vi "Change State.vi"(8 "error in (no error)":errorcluster, 10 "New State":T1=enum."Hover", 11 "Filled Text Fields Actor in":refnum<class "Filled Text Fields Actor.lvclass">) -> (0 "error out":errorcluster, 3 "Filled Text Fields Actor out":refnum<class "Filled Text Fields Actor.lvclass">)   [LabVIEW 2017, in "Filled Text Fields.lvlib" / "Filled Text Fields Actor.lvclass"]
uses:
  Filled Text Fields Actor.lvclass
  Filled Text Fields.States.ctl
  Filled Text Fields Actor.lvclass/Filled Text Fields Actor.ctl
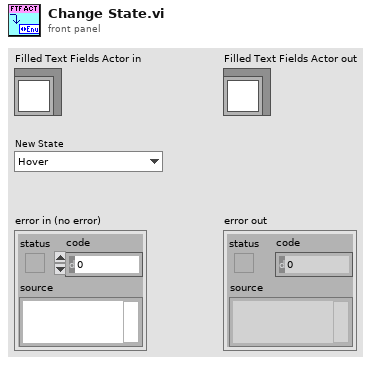
[diagram p1: front panel]
types:
  T1 = typedef "Filled Text Fields.lvlib/Filled Text Fields Actor.lvclass/Filled Text Fields.States.ctl" = enum16{"Inactive", "Activated", "Error", "Focused", "Hover", "Disabled", "Disabled and Grey out"}
  T2 = enum8{"Enabled", "Disabled", "Disabled and Grayed Out"}
  T3 = typedef "Theme.lvlib/Theme.Colors.lvclass/Colors.ctl" = cluster{"Main":cluster{"Primary":u32, "Primary Variant":u32, "Secondary":u32, "Secondary Varient":u32}, "Container":cluster{"BG":u32, "Hover":u32, "Focused":u32}, "Text":cluster{"Default":u32, "Error":u32}}
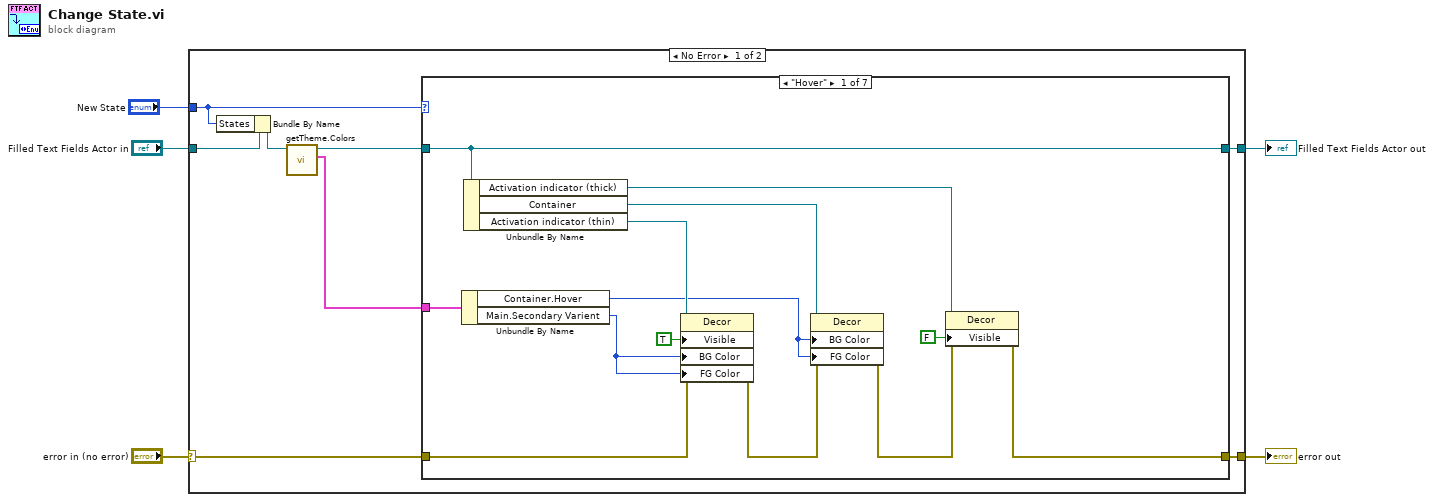
[diagram p0: block diagram]
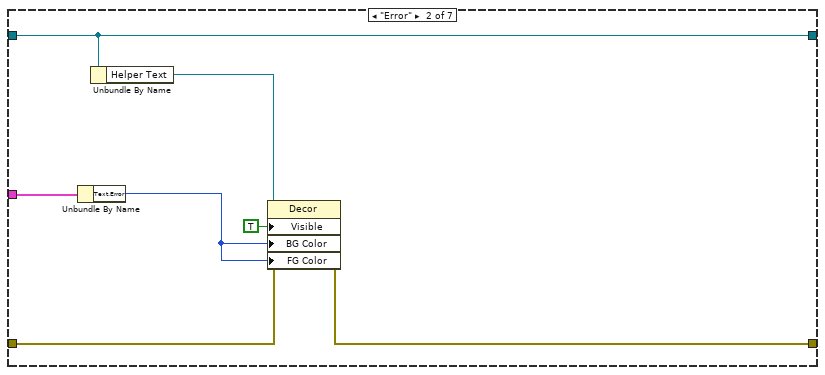
[diagram p2: hidden frame]
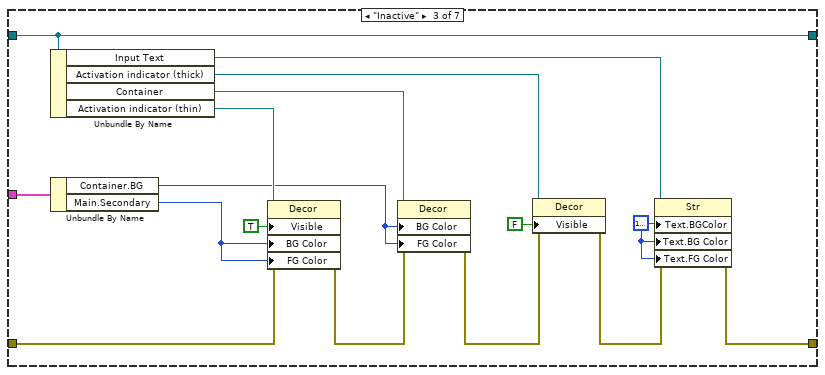
[diagram p3: hidden frame]
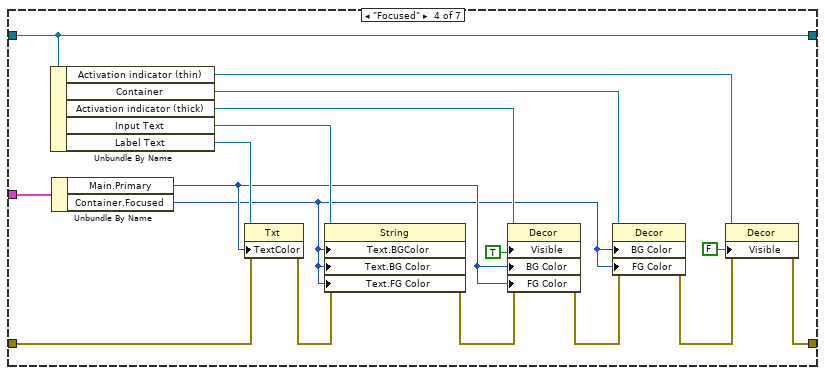
[diagram p4: hidden frame]
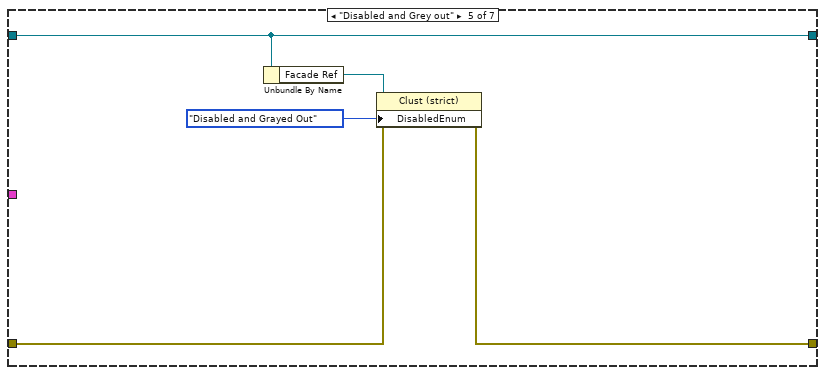
[diagram p5: hidden frame]
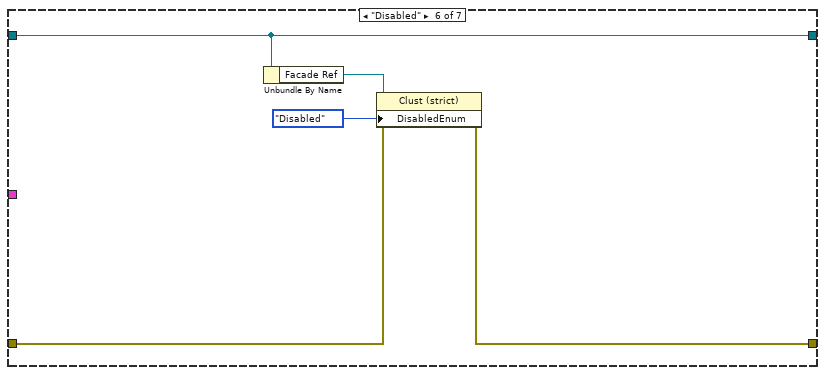
[diagram p6: hidden frame]
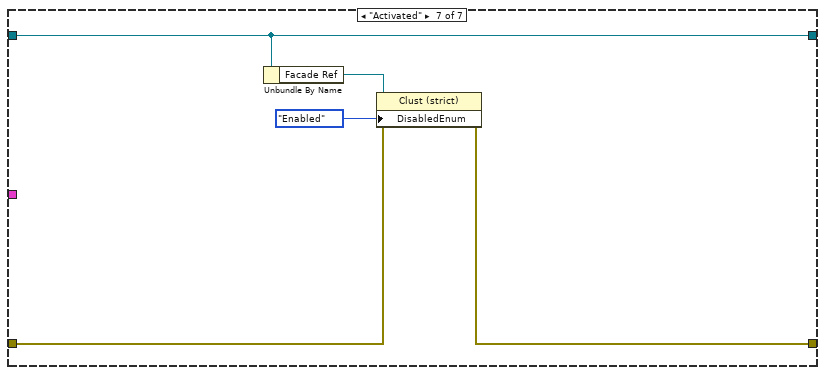
[diagram p7: hidden frame]
diagram:
  n1 = case shown="No Error" "error in (no error)" {
    selector: "error in (no error)" -> [w11 w83]
    tunnel: [w10 w83] -> w4
    tunnel: [w12 w82] -> w2
    tunnel: "Filled Text Fields Actor in" -> [w13 w82]
    tunnel: "New State" -> [w8 _]
    frame No Error {
      n2 = Bundle By Name(cluster=w13, "States"=w8) -> (w9:refnum<class "Filled Text Fields Actor.lvclass">)
      n3 = call "getTheme.Colors.vi"("Filled Text Fields Actor in"=w9) -> ("Colors"=w6:T3, "Filled Text Fields Actor out"=w7:refnum<class "Filled Text Fields Actor.lvclass">)  [unwired: 9 in]
      n4 = case shown="\"Hover\"" w8 {
        tunnel: w7 -> [w22 w32 w45 w62 w71 w76 w81]
        tunnel: [w22 w32 w45 w62 w71 w76 w81] -> w12
        tunnel: w11 -> [w21 w31 w44 w53 w68 w73 w78]
        tunnel: [w18 w29 w38 w59 w67 w72 w77] -> w10
        tunnel: w6 -> [w16 w28 w36 w52 _ _ _]
        frame "Hover" {
          n5 = Unbundle By Name(w16) -> ("Container.Hover"=w14:u32, "Main.Secondary Varient"=w15:u32)
          n6 = Unbundle By Name(w22) -> ("Activation indicator (thick)"=w23:refnum<vi>, "Container"=w25:refnum<vi>, "Activation indicator (thin)"=w17:refnum<vi>)
          n7 = property class="Decor"(reference=w17, error in=w21, "Visible"=TRUE, "BG Color"=w15, "FG Color"=w15) -> (error out=w20:errorcluster)  [unwired: 1 out]
          n8 = property class="Decor"(reference=w25, error in=w20, "BG Color"=w14, "FG Color"=w14) -> (error out=w19:errorcluster)  [unwired: 1 out]
          n9 = property class="Decor"(reference=w23, error in=w19, "Visible"=FALSE) -> (error out=w18:errorcluster)  [unwired: 1 out]
        }
        frame "Error" {
          n10 = Unbundle By Name(w28) -> ("Text.Error"=w27:u32)
          n11 = Unbundle By Name(w32) -> ("Helper Text"=w30:refnum<vi>)
          n12 = property class="Decor"(reference=w30, error in=w31, "Visible"=TRUE, "BG Color"=w27, "FG Color"=w27) -> (error out=w29:errorcluster)  [unwired: 1 out]
        }
        frame "Inactive" {
          w37 = u32 16777216 ("Text.Text Colors:BG Color")
          n13 = Unbundle By Name(w45) -> ("Input Text"=w40:refnum<vi>, "Activation indicator (thick)"=w46:refnum<vi>, "Container"=w48:refnum<vi>, "Activation indicator (thin)"=w41:refnum<vi>)
          n14 = Unbundle By Name(w36) -> ("Container.BG"=w34:u32, "Main.Secondary"=w35:u32)
          n15 = property class="Decor"(reference=w41, error in=w44, "Visible"=TRUE, "BG Color"=w35, "FG Color"=w35) -> (error out=w43:errorcluster)  [unwired: 1 out]
          n16 = property class="Decor"(reference=w48, error in=w43, "BG Color"=w34, "FG Color"=w34) -> (error out=w42:errorcluster)  [unwired: 1 out]
          n17 = property class="Decor"(reference=w46, error in=w42, "Visible"=FALSE) -> (error out=w39:errorcluster)  [unwired: 1 out]
          n18 = property class="Str"(reference=w40, error in=w39, "Text.BGColor"=w37, "Text.BG Color"=w37, "Text.FG Color"=w37) -> (error out=w38:errorcluster)  [unwired: 1 out]
        }
        frame "Focused" {
          n19 = Unbundle By Name(w62) -> ("Activation indicator (thin)"=w63:refnum<vi>, "Container"=w65:refnum<vi>, "Activation indicator (thick)"=w58:refnum<vi>, "Input Text"=w57:refnum<vi>, "Label Text"=w54:refnum<vi>)
          n20 = Unbundle By Name(w52) -> ("Main.Primary"=w51:u32, "Container.Focused"=w50:u32)
          n21 = property class="Txt"(reference=w54, error in=w53, "TextColor"=w51) -> (error out=w55:errorcluster)  [unwired: 1 out]
          n22 = property on="Property Node" class="String"(reference=w57, error in=w55, "Text.BGColor"=w50, "Text.BG Color"=w50, "Text.FG Color"=w50) -> (error out=w56:errorcluster)  [unwired: 1 out]
          n23 = property class="Decor"(reference=w58, error in=w56, "Visible"=TRUE, "BG Color"=w51, "FG Color"=w51) -> (error out=w61:errorcluster)  [unwired: 1 out]
          n24 = property class="Decor"(reference=w65, error in=w61, "BG Color"=w50, "FG Color"=w50) -> (error out=w60:errorcluster)  [unwired: 1 out]
          n25 = property class="Decor"(reference=w63, error in=w60, "Visible"=FALSE) -> (error out=w59:errorcluster)  [unwired: 1 out]
        }
        frame "Disabled and Grey out" {
          n26 = Unbundle By Name(w71) -> ("Facade Ref"=w70:refnum<vi>)
          n27 = property class="Clust (strict)"(reference=w70, error in=w68, "DisabledEnum"=T2."Disabled and Grayed Out" ("Disabled")) -> (error out=w67:errorcluster)  [unwired: 1 out]
        }
        frame "Disabled" {
          n28 = Unbundle By Name(w76) -> ("Facade Ref"=w75:refnum<vi>)
          n29 = property class="Clust (strict)"(reference=w75, error in=w73, "DisabledEnum"=T2."Disabled" ("Disabled")) -> (error out=w72:errorcluster)  [unwired: 1 out]
        }
        frame "Activated" {
          n30 = Unbundle By Name(w81) -> ("Facade Ref"=w80:refnum<vi>)
          n31 = property class="Clust (strict)"(reference=w80, error in=w78, "DisabledEnum"=T2."Enabled" ("Disabled")) -> (error out=w77:errorcluster)  [unwired: 1 out]
        }
      }
    }
    frame Error {
    }
  }
  "error out" <- w4
  "Filled Text Fields Actor out" <- w2
